vi "Instrument AutoScale_EVM (LTE).vi"(0 "Session In":refnum<visa-resource-name>="GPIB0::16::INSTR", 9 "Timeout":u32=3000, 11 "error in":errorcluster {"code" format="%.0x"}, 12 "line index":u16(ring)=1 items=["VECT", "EVM"], 13 "Trace":i32(ring) items=["TRACE1", "TRACE2", "TRACE3", "TRACE4"]) -> (4 "Session Out":refnum<visa-resource-name>="GPIB0::16::INSTR", 15 "error out":errorcluster {"code" format="%.0x"})   [LabVIEW 2018]
doc: "Launches the Instrument I/O Assistant, which you can use to communicate with message-based instruments and graphically parse the response. For example you can communicate with an instrument that uses a serial, Ethernet, or GPIB interface."
panel:
  out "CMD":string=":DISP:VECT:TRAC1:Y:AUTO:ONCE"
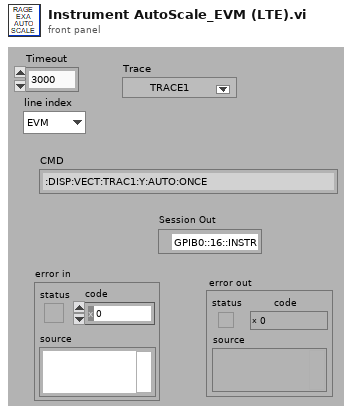
[diagram p1: front panel]
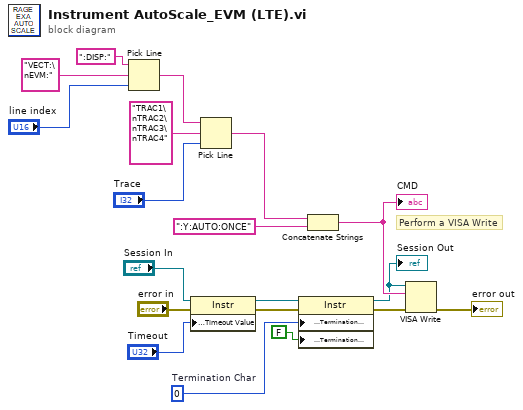
[diagram p0: block diagram]
diagram:
  w14 = u8 0  # Termination Char
  # "Perform a VISA Write"
  n1 = Pick Line(string ("")=":DISP:" ("staticText"), multi-line string="VECT:\nEVM:", line index="line index") -> (output string=w2:string)
  n2 = property class="Instr"(reference="Session In", error in="error in", "General Settings:Timeout Value"="Timeout") -> (reference out=w13:refnum<visa-resource-name>, error out=w16:errorcluster)
  n3 = Pick Line(string ("")=w2, multi-line string="TRAC1\nTRAC2\nTRAC3\nTRAC4", line index="Trace") -> (output string=w1:string)
  n4 = property class="Instr"(reference=w13, error in=w16, "Message Based Settings:Termination Character"=w14, "Message Based Settings:Termination Character Enable"=FALSE ("enable")) -> (reference out=w8:refnum<visa-resource-name>, error out=w15:errorcluster)
  "Session Out" <- w8
  n5 = Concatenate Strings(w1, ":Y:AUTO:ONCE" ("StaticText")) -> (w10:string)
  "CMD" <- w10
  n6 = VISA Write(VISA resource name=w8, write buffer=w10, error in (no error)=w15) -> (error out=→"error out":errorcluster)  [unwired: 2 out]
